vi "CH_LM Test SCPI.vi"() -> ()   [LabVIEW 2012, in "CH_LM.lvlib"]
doc: "This example VI can be used to execute SCPI commands manually."
uses:
  CH_LM.lvlib
  CH_LM/CH_LM BaudRates.ctl
  CH_LM/CH_LM Parity.ctl
  CH_LM/CH_LM SerialConfiguration.ctl
panel:
  in  "Serial Configuration\n(19200,N,8,1)":T1={"Baud Rate"=19200, "Parity"=0, "Data Bits"=8, "Stop Bits"=1} {"Parity" items=["None", "Odd", "Even"]; "Baud Rate" items=["9600"=9600, "19200"=19200, "38400"=38400, "57600"=57600, "115200"=115200]}
  in  "send SCPI":bool
  out "Response Array":string[](array[string])
  out "Response":string
  in  "NofStrings (-1:all)":i32=-1
  in  "SCPI Command/Query":string
  out "stopped":bool
  out "loop":i32
  in  "Reset":bool
  out "error out":errorcluster
  in  "stop":bool
  out "timed out?":bool
  in  "Address":i32=1
  in  "Serial Number":string
  in  "Reset? (F: No)":bool
  in  "ID Query? (T: Yes)":bool
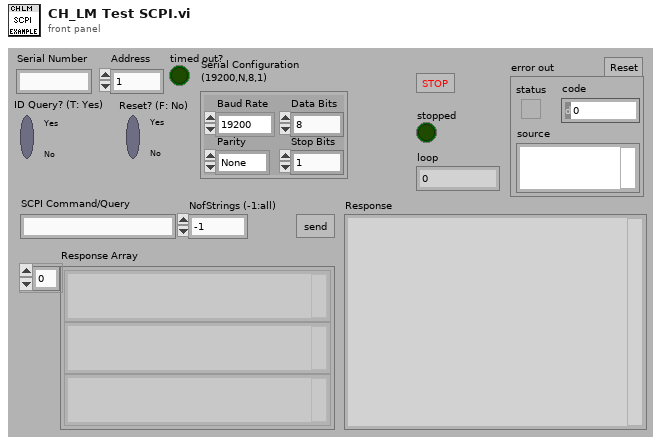
[diagram p1: front panel]
types:
  T1 = typedef "CH_LM.lvlib/CH_LM SerialConfiguration.ctl" = cluster{"Baud Rate":T2, "Parity":T3, "Data Bits":u16, "Stop Bits":u16}
  T2 = typedef "CH_LM.lvlib/CH_LM BaudRates.ctl" = u32
  T3 = typedef "CH_LM.lvlib/CH_LM Parity.ctl" = u16
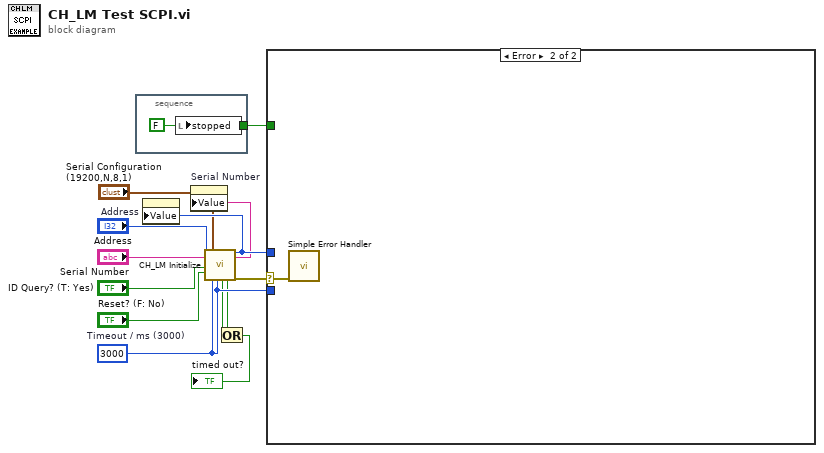
[diagram p0: block diagram]
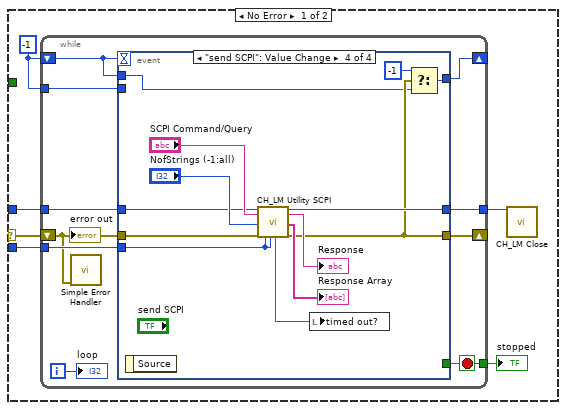
[diagram p2: hidden frame]
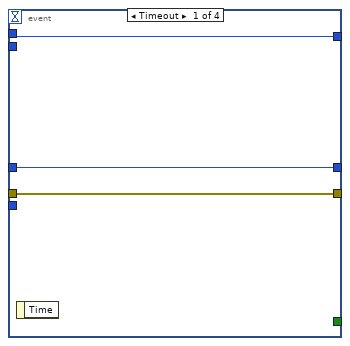
[diagram p3: hidden frame]
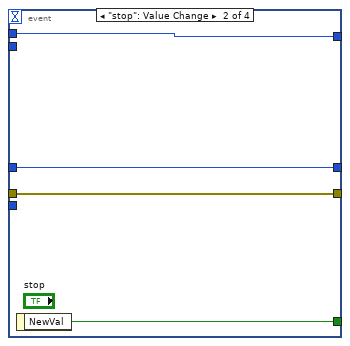
[diagram p4: hidden frame]
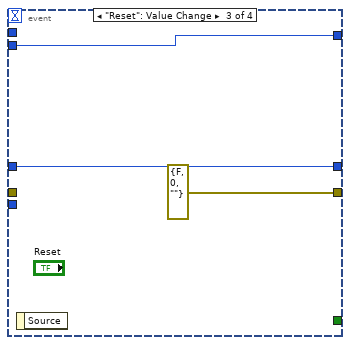
[diagram p5: hidden frame]
diagram:
  w10 = 3000  # Timeout / ms (3000)
  n1 = stacked-sequence {
    tunnel: [w14] -> w7
    frame #0 {
      w14 = FALSE ("stopped")
      n2 = local write "stopped"(w14) -> ()
    }
  }
  n3 = call "CH_LM Initialize.vi"("Address"="Address", "Serial Number"="Serial Number", "ID Query (True)"="ID Query? (T: Yes)", "Reset (False)"="Reset? (F: No)", "Serial Configuration\n(19200,N,8,1)"="Serial Configuration\n(19200,N,8,1)", "Timeout / ms (3000)"=w10, "Lock Timeout / ms (1000)"=w10) -> ("Lock timed out"=w9:bool, "timed out?"=w8:bool, "Meter Index"=w3:i32, "Serial Number"=w2:string, "error out"=w11:errorcluster)  [unwired: 1 in, 7 out]
  n4 = property on="Address" class="DigNum (strict)"("Value"=w3) -> ()  [unwired: 2 in, 2 out]
  n5 = property on="Serial Number" class="Str"("Value"=w2) -> ()  [unwired: 2 in, 2 out]
  n6 = Or(x=w8, y=w9) -> (x .or. y?=→"timed out?":bool)
  n7 = case shown="Error" w11 {
    selector: w11 -> [w15 w54]
    tunnel: w3 -> [w16 _]
    tunnel: w10 -> [w17 _]
    tunnel: w7 -> [_ _]
    frame No Error {
      w18 = -1
      n8 = while {
        tunnel: w16 -> [w30]
        tunnel: [w29] -> w20
        shift-right: [w28] -> _
        shift-left: w15 -> [w22]
        tunnel: w17 -> [w27]
        tunnel: [w25] -> w19
        shift-right: [w24] -> _
        shift-left: w18 -> [w21]
        tunnel: w18 -> [w23]
        i -> [w26]
        stop <- w25 stop-if-true
        n9 = call <vilib>:"Simple Error Handler.vi"("error in (no error)"=w22) -> ()  [unwired: 1 in, 8 out]
        n10 = event shown="[3] \"send SCPI\": Value Change" {
          selector: _ -> [_ _ _ _]
          dyn-events: _ -> [_ _ _ _]
          timeout: w21 -> [_ _ _ _]
          tunnel: [_ w37 _ _] -> w25
          tunnel: w30 -> [w31 w36 w39 w49]
          tunnel: w22 -> [w33 w35 _ w48]
          tunnel: [w31 w36 w39 w46] -> w29
          tunnel: [w33 w35 errorcluster {"status"=FALSE, "code"=0, "source"=""} ("error out") w45] -> w28
          tunnel: w27 -> [_ _ _ w47]
          tunnel: [w32 w34 w38 w44] -> w24
          tunnel: w23 -> [_ _ w38 _]
          tunnel: w21 -> [w32 w34 _ w42]
          event Timeout {
            n11 = event-data() -> ()  [unwired: 2 out]
          }
          event "stop": Value Change {
            n12 = event-data() -> ("NewVal"=w37:bool)  [unwired: 1 out]
          }
          event "Reset": Value Change {
            n13 = event-data() -> ()  [unwired: 2 out]
          }
          event "send SCPI": Value Change {
            n14 = event-data() -> ()  [unwired: 2 out]
            n15 = call "CH_LM Utility SCPI.vi"("Meter Index"=w49, "SCPI Command/Query"="SCPI Command/Query", "NofStrings (-1:all)"="NofStrings (-1:all)", "error in (no error)"=w48, "Timeout / ms (3000)"=w47, "Lock Timeout / ms (1000)"=w47) -> ("Lock timed out"=w41:bool, "Meter Index"=w46:i32, "Response"=→"Response":string, "Response Array"=→"Response Array":string[], "error out"=w45:errorcluster)  [unwired: 9 out]
            n16 = local write "timed out?"(w41) -> ()
            n17 = Select(t=-1, s=w45, f=w42) -> (s? t:f=w44:i32)
          }
        }
        "error out" <- w22
        "loop" <- w26
      }
      "stopped" <- w19
      n18 = call "CH_LM Close.vi"("Meter Index"=w20) -> ()  [unwired: 1 in, 18 out]
    }
    frame Error {
      n19 = call <vilib>:"Simple Error Handler.vi"("error in (no error)"=w54) -> ()  [unwired: 1 in, 8 out]
    }
  }
